vi "Write Device ID.vi"(8 "error in (no error)":errorcluster, 10 "Device ID":string, 11 "Send Data Msg in":refnum<class "Send Data Msg.lvclass">) -> (0 "error out":errorcluster, 3 "Send Data Msg out":refnum<class "Send Data Msg.lvclass">)   [LabVIEW 2014, in "Send Data Msg.lvclass"]
uses:
  Send Data Msg.lvclass
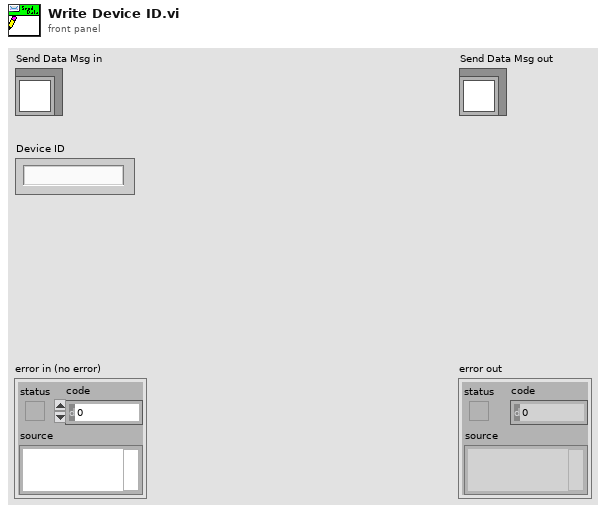
[diagram p1: front panel]
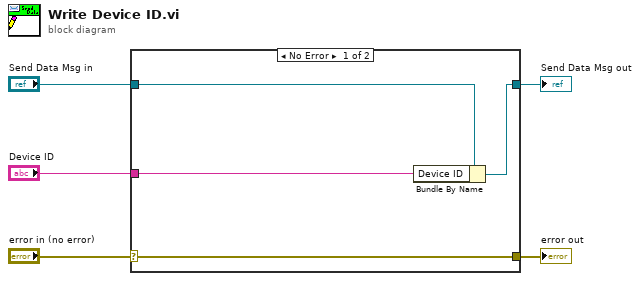
[diagram p0: block diagram]
diagram:
  n1 = case shown="No Error" "error in (no error)" {
    selector: "error in (no error)" -> [w9 w10]
    tunnel: [w9 w10] -> w4
    tunnel: [w7 w11] -> w2
    tunnel: "Send Data Msg in" -> [w8 w11]
    tunnel: "Device ID" -> [w6 _]
    frame No Error {
      n2 = Bundle By Name(cluster=w8, "Device ID"=w6) -> (w7:refnum<class "Send Data Msg.lvclass">)
    }
    frame Error {
    }
  }
  "error out" <- w4
  "Send Data Msg out" <- w2
